vi "centroid_light field correction.vi"(10 "ROI array (no trans)":u8[][](array[numeric])) -> (1 "xybase core":i32, 3 "ROI array out":u8[][](array[numeric]))   [LabVIEW 2017]
doc: "本VI的功能是对图心的搜索进行亮场修正。图心算法十分高效，但是对背景光十分敏感，背景光会导致图心位置偏移，因此，本VI找出ROI区域的亮度中值视为背景光的均值，然后ROI中所有强度值减去中值，再取绝对值，这样就完美地加强了偏离背景光较大的衍射环图案在图心计算中的权重。"
uses:
  <vilib>/Analysis/NI_AALBase.lvlib
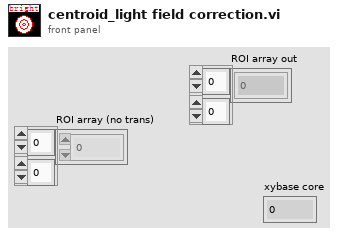
[diagram p1: front panel]
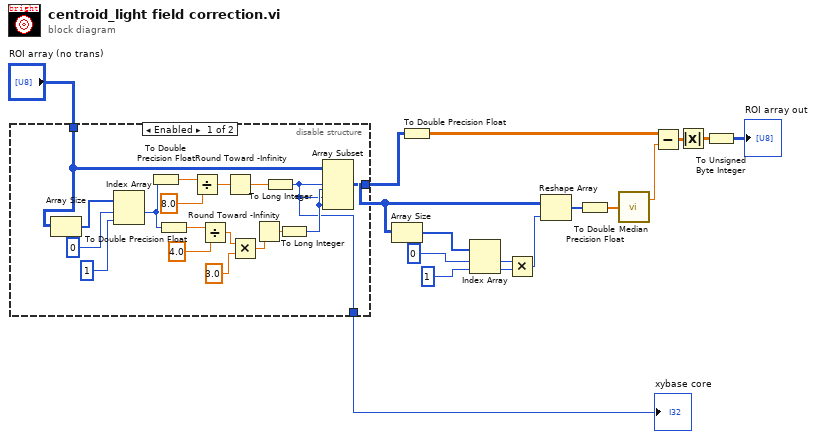
[diagram p0: block diagram]
diagram:
  n1 = disable-structure shown="Enabled" {
    disable-tunnel: [w22 _] -> w4
    disable-tunnel: "ROI array (no trans)" -> [w21 w35]
    disable-tunnel: [w17 w35] -> w1
    frame Enabled {
      n2 = Array Size(array=w21) -> (size(s)=w32:i32[])
      n3 = Index Array(array=w32, index #1=0 ("索引"), index #2=1 ("索引")) -> (element #1=w24:i32)  [unwired: 1 out]
      n4 = To Double Precision Float(number=w24) -> (double precision float=w31:dbl)
      n5 = To Double Precision Float(number=w24) -> (double precision float=w25:dbl)
      n6 = Divide(x=w31, y=8.0) -> (x/y=w29:dbl)
      n7 = Divide(x=w25, y=4.0) -> (x/y=w20:dbl)
      n8 = Round Toward -Infinity(1:w29) -> (0:w28:dbl)
      n9 = Multiply(x=w20, y=3.0) -> (x*y=w18:dbl)
      n10 = Round Toward -Infinity(1:w18) -> (0:w27:dbl)
      n11 = To Long Integer(number=w28) -> (32bit integer=w22:i32)
      n12 = To Long Integer(number=w27) -> (32bit integer=w23:i32)
      n13 = Array Subset(array=w21, index (row)=w22, length (row)=w23, index (col)=w22, length (col)=w23) -> (w17:u8[][])
    }
    frame Disabled {
    }
  }
  "xybase core" <- w4
  n14 = Array Size(array=w1) -> (size(s)=w11:i32[])
  n15 = To Double Precision Float(number=w1) -> (double precision float=w13:dbl[][])
  n16 = Index Array(array=w11, index #1=0 ("索引"), index #2=1 ("索引")) -> (element #1=w7:i32, element #2=w8:i32)
  n17 = Multiply(x=w7, y=w8) -> (x*y=w6:i32)
  n18 = Reshape Array(w1, w6) -> (w15:u8[])
  n19 = To Double Precision Float(number=w15) -> (double precision float=w16:dbl[])
  n20 = call <vilib>:"Median.vi"("X"=w16) -> ("median"=w14:dbl)  [unwired: 1 out]
  n21 = Subtract(x=w13, y=w14) -> (x-y=w5:dbl[][])
  n22 = Absolute Value(x=w5) -> (abs(x)=w12:dbl[][])
  n23 = To Unsigned Byte Integer(number=w12) -> (unsigned 8bit integer=→"ROI array out":u8[][])
